vi "Sort By Name.vi"(10 "Panel B":refnum<class "Panel.lvclass">, 11 "Panel A":refnum<class "Panel.lvclass">) -> (3 "A < B":bool)   [LabVIEW 2020, in "PicoG-App.lvlib" / "AppListPanel.lvclass"]
uses:
  AppListPanel.lvclass
  GWebAppArrayPanel/GWebAppArrayPanel.lvclass
  ViaApp/ViaApp.lvclass
  <vilib>/IlluminatedG/IG OOPanel/OOPanel/Panel/Panel.lvclass
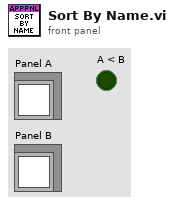
[diagram p1: front panel]
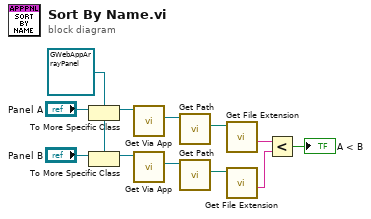
[diagram p0: block diagram]
diagram:
  w12 = refnum<class "GWebAppArrayPanel.lvclass"> refnum ("PicoG-App.lvlib:GWebAppArrayPanel.lvclass")
  n1 = To More Specific Class(target class=w12, reference="Panel A") -> (specific class reference=w11:refnum<class "GWebAppArrayPanel.lvclass">)  [unwired: 1 in, 1 out]
  n2 = To More Specific Class(target class=w12, reference="Panel B") -> (specific class reference=w10:refnum<class "GWebAppArrayPanel.lvclass">)  [unwired: 1 in, 1 out]
  n3 = call "Get Via App.vi"("GWebAppArrayPanel in"=w11) -> ("App"=w7:refnum<class "ViaApp.lvclass">)  [unwired: 8 in, 2 out]
  n4 = call "Get Via App.vi"("GWebAppArrayPanel in"=w10) -> ("App"=w6:refnum<class "ViaApp.lvclass">)  [unwired: 8 in, 2 out]
  n5 = call "Get Path.vi"("ViaApp in"=w7) -> ("Path"=w4:path)  [unwired: 8 in, 2 out]
  n6 = call "Get Path.vi"("ViaApp in"=w6) -> ("Path"=w5:path)  [unwired: 8 in, 2 out]
  n7 = call <vilib>:"Get File Extension.vi"("file"=w4) -> ("filename without extension"=w3:string)  [unwired: 6 in, 4 out]
  n8 = call <vilib>:"Get File Extension.vi"("file"=w5) -> ("filename without extension"=w2:string)  [unwired: 6 in, 4 out]
  n9 = Less?(x=w3, y=w2) -> (x < y?=→"A < B":bool)
